vi "Parse.vi"(8 "Error In":errorcluster, 11 "object in":refnum<class "2022_5.lvclass">) -> (0 "Error Out":errorcluster, 3 "object out":refnum<class "2022_5.lvclass">)   [LabVIEW 2020, in "2022_5.lvclass"]
uses:
  2022_5.lvclass
  2022_5.lvclass/2022_5.ctl
  3533d167-0fa0-486d-894b-d8c4a5850acb.vi
  3533d167-0fa0-486d-894b-d8c4a5850acb.vi/be6f088c-3e4b-4523-ad48-2cdc85bad38a.vi
  3533d167-0fa0-486d-894b-d8c4a5850acb.vi/f202eadf-433e-4cdb-b986-b2351ce8d73c.vi
  3533d167-0fa0-486d-894b-d8c4a5850acb.vi/094751bc-bcf2-4346-afae-53942128b536.vi
panel:
  out "Stacks":cluster{"Crates":string[]}[](array[cluster])
  out "Stacks 2":string[][](array[string])
  out "Stacks":string[][](array[string])
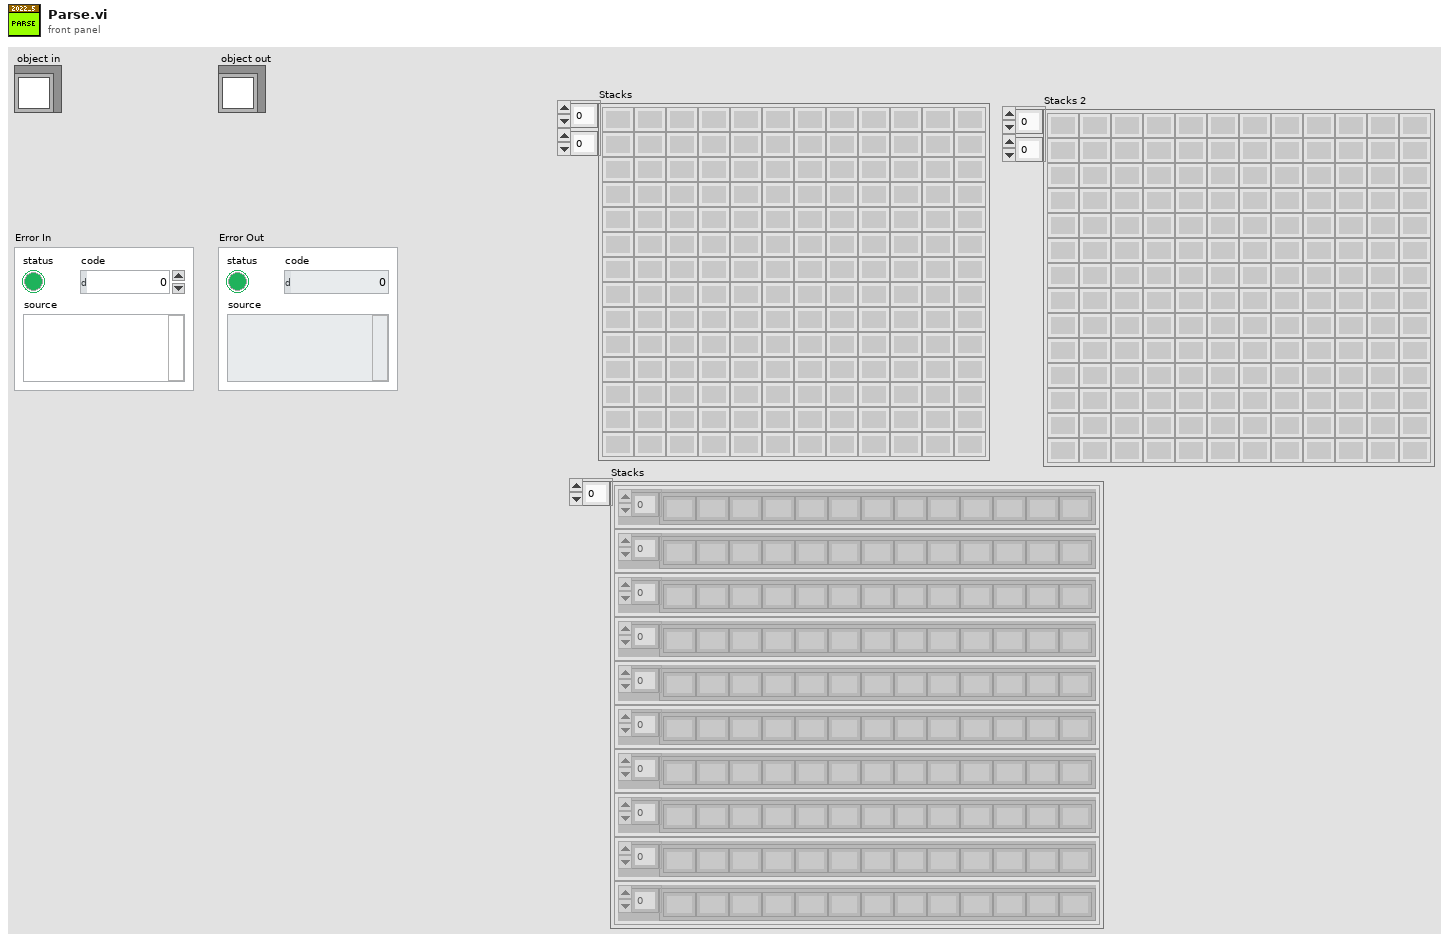
[diagram p1: front panel]
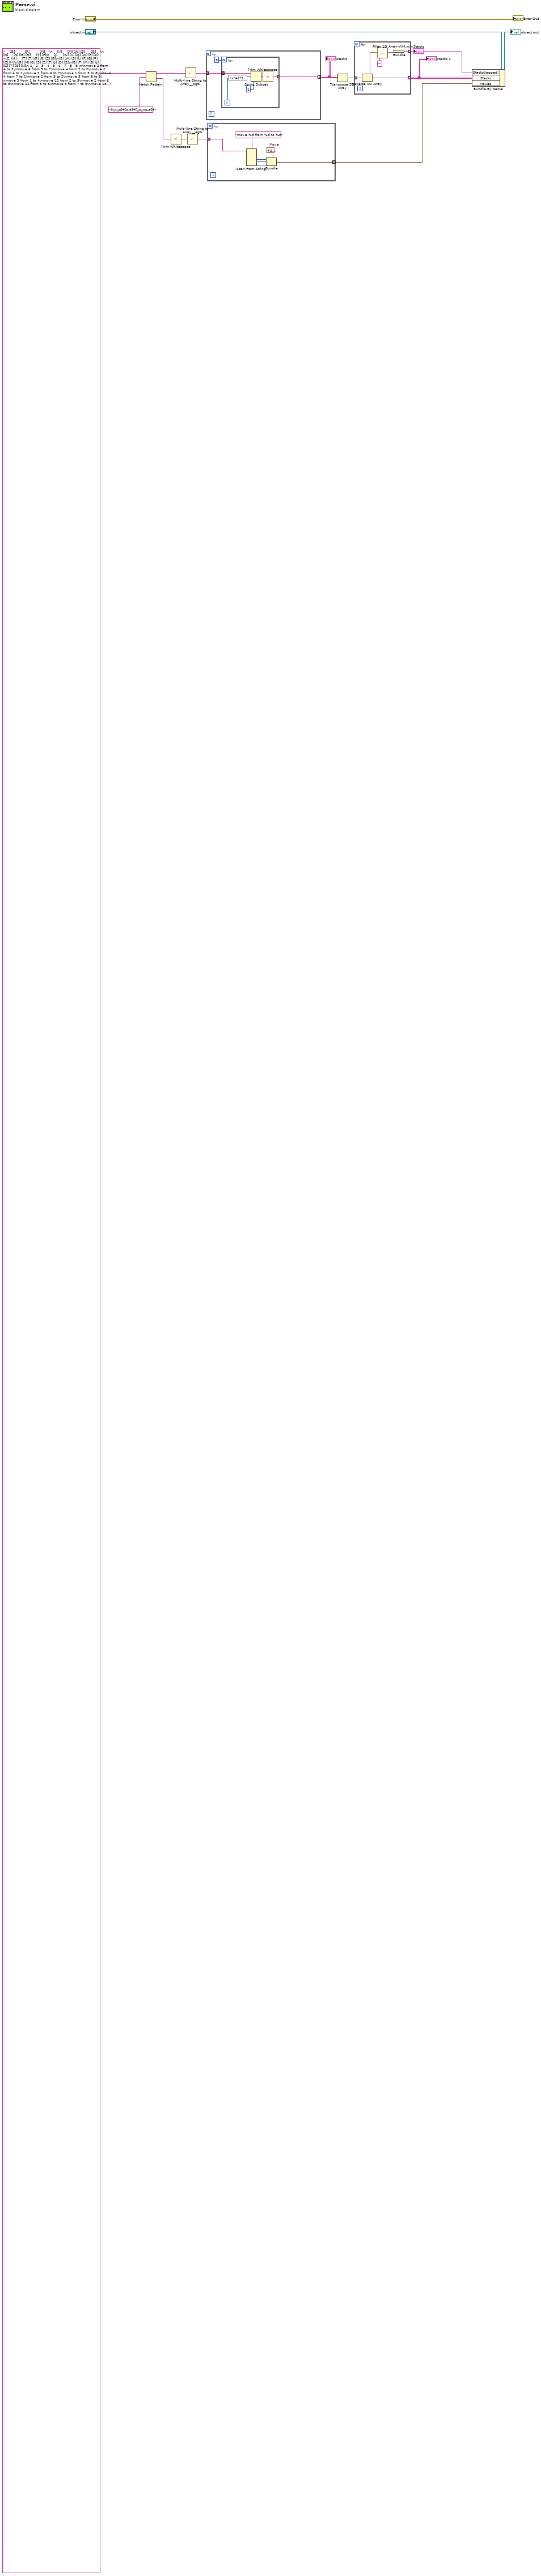
[diagram p0: block diagram]
diagram:
  n1 = Match Pattern(string="    [G]         [P]         [M]    \n    [V]     [M] [W] [S]     [Q]    \n    [N]     [N] [G] [H]     [T] [F]\n    [J]     [W] [V] [Q] [W] [F] [P]\n[C] [H]     [T] [T] [G] [B] [Z] [B]\n[S] [W] [S] [L] [F] [B] [P] [C] [H]\n[G] [M] [Q] [S] [Z] [T] [J] [D] [S]\n[B] [T] [M] [B] [J] [C] [T] [G] [N]\n 1   2   3   4   5   6   7   8   9 \n\nmove 2 from 4 to 2\nmove 6 from 9 to 7\nmove 4 from 7 to 2\nmove 2 from 4 to 1\nmove 2 from 6 to 7\nmove 1 from 3 to 8\nmove 4 from 7 to 1\nmove 2 from 3 to 2\nmove 3 from 8 to 5\nmove 3 from 1 to 4\nmove 12 from 2 to 5\nmove 2 from 6 to 8\nmove 12 from 5 to 8\nmove 3 from 7 to 9\nmove 18 from 8 to 9\nmove 2 from 8 to 6\nmove 3 from 2 to 3\nmove 14 from 9 to 4\nmove 1 from 1 to 3\nmove 7 from 9 to 3\nmove 1 from 2 to 1\nmove 8 from 4 to 5\nmove 5 from 6 to 3\nmove 2 from 7 to 9\nmove 3 from 4 to 9\nmove 4 from 9 to 6\nmove 4 from 6 to 1\nmove 8 from 4 to 6\nmove 10 from 1 to 2\nmove 13 from 3 to 2\nmove 17 from 5 to 9\nmove 2 from 5 to 1\nmove 9 from 9 to 7\nmove 1 from 3 to 6\nmove 2 from 1 to 8\nmove 11 from 2 to 4\nmove 5 from 6 to 8\nmove 1 from 6 to 3\nmove 1 from 1 to 4\nmove 3 from 8 to 6\nmove 3 from 2 to 8\nmove 9 from 7 to 9\nmove 4 from 4 to 7\nmove 1 from 9 to 5\nmove 15 from 9 to 7\nmove 7 from 8 to 3\nmove 1 from 5 to 6\nmove 2 from 6 to 9\nmove 8 from 2 to 6\nmove 3 from 4 to 3\nmove 1 from 2 to 5\nmove 4 from 9 to 3\nmove 1 from 3 to 4\nmove 13 from 6 to 2\nmove 1 from 5 to 1\nmove 4 from 4 to 9\nmove 6 from 3 to 2\nmove 11 from 2 to 7\nmove 6 from 3 to 4\nmove 3 from 3 to 2\nmove 1 from 3 to 4\nmove 1 from 1 to 3\nmove 3 from 9 to 2\nmove 1 from 3 to 1\nmove 4 from 7 to 1\nmove 1 from 9 to 5\nmove 5 from 1 to 4\nmove 11 from 2 to 4\nmove 1 from 5 to 3\nmove 1 from 2 to 3\nmove 12 from 4 to 2\nmove 2 from 7 to 2\nmove 7 from 4 to 3\nmove 5 from 4 to 1\nmove 7 from 7 to 6\nmove 4 from 1 to 8\nmove 1 from 8 to 5\nmove 8 from 3 to 2\nmove 4 from 7 to 4\nmove 13 from 7 to 1\nmove 2 from 8 to 6\nmove 5 from 4 to 9\nmove 1 from 3 to 6\nmove 1 from 5 to 8\nmove 1 from 2 to 9\nmove 4 from 2 to 6\nmove 2 from 8 to 6\nmove 10 from 1 to 3\nmove 4 from 9 to 4\nmove 2 from 1 to 3\nmove 5 from 2 to 9\nmove 4 from 9 to 2\nmove 1 from 1 to 2\nmove 13 from 2 to 4\nmove 15 from 4 to 5\nmove 3 from 6 to 8\nmove 8 from 3 to 8\nmove 1 from 4 to 2\nmove 14 from 5 to 1\nmove 1 from 5 to 4\nmove 1 from 4 to 2\nmove 8 from 6 to 7\nmove 3 from 6 to 2\nmove 2 from 9 to 1\nmove 8 from 8 to 7\nmove 9 from 1 to 5\nmove 7 from 5 to 3\nmove 14 from 7 to 9\nmove 2 from 2 to 3\nmove 7 from 2 to 1\nmove 1 from 6 to 1\nmove 4 from 9 to 2\nmove 8 from 3 to 6\nmove 2 from 4 to 3\nmove 4 from 3 to 5\nmove 5 from 5 to 7\nmove 2 from 6 to 9\nmove 6 from 6 to 2\nmove 4 from 2 to 3\nmove 1 from 6 to 2\nmove 2 from 7 to 8\nmove 13 from 9 to 5\nmove 2 from 7 to 1\nmove 14 from 1 to 5\nmove 15 from 5 to 7\nmove 3 from 8 to 7\nmove 5 from 3 to 5\nmove 6 from 5 to 7\nmove 4 from 1 to 7\nmove 1 from 2 to 5\nmove 3 from 2 to 8\nmove 11 from 5 to 2\nmove 10 from 7 to 1\nmove 1 from 3 to 4\nmove 10 from 2 to 9\nmove 1 from 5 to 8\nmove 6 from 7 to 3\nmove 1 from 4 to 6\nmove 2 from 3 to 8\nmove 1 from 2 to 1\nmove 4 from 3 to 9\nmove 3 from 1 to 6\nmove 2 from 7 to 1\nmove 1 from 5 to 6\nmove 1 from 3 to 8\nmove 4 from 1 to 4\nmove 5 from 2 to 9\nmove 3 from 1 to 4\nmove 18 from 9 to 7\nmove 4 from 8 to 4\nmove 3 from 1 to 2\nmove 1 from 9 to 7\nmove 1 from 4 to 7\nmove 1 from 6 to 2\nmove 1 from 2 to 5\nmove 25 from 7 to 3\nmove 7 from 4 to 2\nmove 8 from 7 to 9\nmove 4 from 8 to 6\nmove 1 from 8 to 5\nmove 4 from 6 to 5\nmove 2 from 9 to 5\nmove 3 from 5 to 8\nmove 4 from 6 to 4\nmove 12 from 3 to 5\nmove 11 from 3 to 2\nmove 13 from 5 to 8\nmove 4 from 9 to 6\nmove 7 from 4 to 9\nmove 2 from 6 to 2\nmove 12 from 2 to 7\nmove 1 from 6 to 3\nmove 1 from 5 to 6\nmove 2 from 5 to 3\nmove 15 from 8 to 6\nmove 4 from 6 to 7\nmove 1 from 5 to 1\nmove 10 from 2 to 8\nmove 8 from 8 to 3\nmove 8 from 6 to 8\nmove 2 from 7 to 6\nmove 9 from 9 to 7\nmove 8 from 8 to 9\nmove 1 from 1 to 3\nmove 1 from 2 to 7\nmove 7 from 3 to 1\nmove 3 from 8 to 5\nmove 3 from 1 to 6\nmove 7 from 9 to 2\nmove 2 from 3 to 7\nmove 5 from 7 to 9\nmove 17 from 7 to 5\nmove 2 from 7 to 6\nmove 10 from 6 to 3\nmove 1 from 1 to 3\nmove 6 from 9 to 3\nmove 1 from 2 to 9\nmove 2 from 7 to 9\nmove 2 from 9 to 7\nmove 1 from 5 to 8\nmove 1 from 8 to 5\nmove 6 from 2 to 5\nmove 1 from 6 to 1\nmove 5 from 3 to 5\nmove 1 from 6 to 8\nmove 1 from 7 to 9\nmove 2 from 9 to 3\nmove 15 from 5 to 2\nmove 2 from 1 to 8\nmove 2 from 3 to 7\nmove 2 from 8 to 3\nmove 3 from 5 to 9\nmove 1 from 8 to 6\nmove 1 from 9 to 6\nmove 3 from 7 to 6\nmove 17 from 3 to 4\nmove 1 from 1 to 2\nmove 6 from 2 to 9\nmove 16 from 4 to 1\nmove 4 from 6 to 8\nmove 9 from 5 to 6\nmove 8 from 6 to 2\nmove 2 from 9 to 5\nmove 2 from 3 to 5\nmove 1 from 6 to 2\nmove 1 from 4 to 8\nmove 14 from 1 to 3\nmove 8 from 5 to 3\nmove 20 from 3 to 1\nmove 1 from 8 to 2\nmove 1 from 9 to 6\nmove 1 from 6 to 7\nmove 1 from 7 to 3\nmove 22 from 1 to 2\nmove 3 from 3 to 6\nmove 27 from 2 to 8\nmove 2 from 2 to 8\nmove 2 from 6 to 9\nmove 2 from 9 to 4\nmove 2 from 4 to 8\nmove 1 from 1 to 3\nmove 14 from 8 to 5\nmove 1 from 3 to 9\nmove 3 from 9 to 2\nmove 5 from 2 to 8\nmove 10 from 2 to 9\nmove 1 from 6 to 7\nmove 1 from 7 to 5\nmove 7 from 5 to 2\nmove 2 from 9 to 2\nmove 1 from 6 to 2\nmove 2 from 9 to 5\nmove 3 from 5 to 6\nmove 6 from 5 to 3\nmove 1 from 5 to 6\nmove 4 from 3 to 9\nmove 2 from 9 to 8\nmove 3 from 9 to 5\nmove 23 from 8 to 1\nmove 2 from 6 to 1\nmove 1 from 5 to 7\nmove 2 from 3 to 5\nmove 2 from 9 to 5\nmove 4 from 9 to 7\nmove 2 from 9 to 4\nmove 1 from 5 to 4\nmove 5 from 8 to 5\nmove 2 from 6 to 2\nmove 3 from 7 to 3\nmove 1 from 3 to 4\nmove 3 from 2 to 8\nmove 4 from 1 to 6\nmove 2 from 6 to 3\nmove 4 from 1 to 2\nmove 3 from 8 to 1\nmove 13 from 2 to 5\nmove 4 from 3 to 2\nmove 14 from 5 to 7\nmove 5 from 2 to 7\nmove 18 from 7 to 9\nmove 4 from 4 to 7\nmove 2 from 5 to 4\nmove 17 from 9 to 5\nmove 1 from 9 to 1\nmove 1 from 7 to 2\nmove 5 from 7 to 2\nmove 18 from 1 to 4\nmove 1 from 7 to 3\nmove 1 from 3 to 6\nmove 2 from 1 to 3\nmove 1 from 6 to 5\nmove 2 from 6 to 8\nmove 1 from 8 to 9\nmove 1 from 8 to 3\nmove 13 from 4 to 5\nmove 1 from 1 to 6\nmove 3 from 2 to 4\nmove 1 from 6 to 1\nmove 3 from 2 to 9\nmove 3 from 3 to 1\nmove 5 from 4 to 5\nmove 30 from 5 to 3\nmove 1 from 4 to 6\nmove 1 from 9 to 8\nmove 1 from 9 to 6\nmove 21 from 3 to 7\nmove 3 from 1 to 6\nmove 1 from 1 to 4\nmove 1 from 9 to 6\nmove 1 from 8 to 2\nmove 1 from 3 to 6\nmove 1 from 9 to 3\nmove 5 from 4 to 8\nmove 1 from 2 to 4\nmove 9 from 5 to 7\nmove 2 from 5 to 9\nmove 2 from 8 to 2\nmove 2 from 6 to 3\nmove 1 from 4 to 1\nmove 4 from 3 to 8\nmove 2 from 9 to 2\nmove 4 from 2 to 6\nmove 1 from 1 to 4\nmove 2 from 6 to 9\nmove 2 from 5 to 4\nmove 1 from 3 to 1\nmove 1 from 1 to 3\nmove 2 from 9 to 1\nmove 5 from 3 to 5\nmove 1 from 1 to 8\nmove 4 from 6 to 4\nmove 5 from 5 to 6\nmove 18 from 7 to 5\nmove 1 from 3 to 4\nmove 12 from 7 to 5\nmove 15 from 5 to 6\nmove 1 from 5 to 8\nmove 1 from 3 to 7\nmove 1 from 1 to 2\nmove 1 from 2 to 4\nmove 1 from 7 to 9\nmove 2 from 8 to 2\nmove 1 from 2 to 4\nmove 4 from 4 to 2\nmove 1 from 2 to 1\nmove 1 from 9 to 8\nmove 4 from 6 to 4\nmove 3 from 2 to 6\nmove 1 from 2 to 6\nmove 8 from 4 to 3\nmove 1 from 1 to 3\nmove 6 from 6 to 1\nmove 1 from 3 to 6\nmove 5 from 1 to 7\nmove 10 from 5 to 9\nmove 3 from 9 to 8\nmove 7 from 6 to 2\nmove 1 from 7 to 8\nmove 3 from 5 to 8\nmove 3 from 6 to 2\nmove 6 from 8 to 9\nmove 1 from 5 to 3\nmove 2 from 3 to 1\nmove 2 from 4 to 8\nmove 6 from 6 to 9\nmove 1 from 1 to 4\nmove 17 from 9 to 2\nmove 1 from 4 to 1\nmove 2 from 7 to 8\nmove 1 from 9 to 8\nmove 3 from 8 to 4\nmove 3 from 1 to 4\nmove 9 from 8 to 2\nmove 1 from 8 to 4\nmove 12 from 2 to 7\nmove 4 from 7 to 4\nmove 1 from 8 to 1\nmove 10 from 4 to 2\nmove 3 from 3 to 2\nmove 1 from 9 to 7\nmove 11 from 7 to 3\nmove 1 from 3 to 1\nmove 2 from 3 to 9\nmove 1 from 3 to 7\nmove 2 from 1 to 9\nmove 1 from 6 to 5\nmove 7 from 3 to 6\nmove 1 from 7 to 3\nmove 3 from 3 to 4\nmove 1 from 5 to 7\nmove 2 from 4 to 3\nmove 2 from 4 to 8\nmove 1 from 7 to 6\nmove 2 from 6 to 8\nmove 1 from 9 to 2\nmove 1 from 9 to 5\nmove 1 from 5 to 1\nmove 1 from 8 to 6\nmove 1 from 3 to 2\nmove 4 from 6 to 1\nmove 5 from 1 to 4\nmove 11 from 2 to 4\nmove 2 from 8 to 2\nmove 1 from 8 to 9\nmove 27 from 2 to 5\nmove 4 from 6 to 3\nmove 3 from 2 to 4\nmove 2 from 5 to 9\nmove 1 from 5 to 7\nmove 2 from 9 to 5\nmove 14 from 4 to 7\nmove 2 from 4 to 7\nmove 3 from 4 to 8\nmove 4 from 3 to 1\nmove 4 from 1 to 8\nmove 2 from 3 to 9\nmove 2 from 9 to 3\nmove 7 from 8 to 9\nmove 1 from 3 to 8\nmove 2 from 3 to 2\nmove 25 from 5 to 9\nmove 1 from 5 to 8\nmove 1 from 8 to 7\nmove 26 from 9 to 1\nmove 23 from 1 to 5\nmove 7 from 9 to 7\nmove 1 from 9 to 8\nmove 1 from 9 to 2\nmove 5 from 7 to 1\nmove 20 from 5 to 6\nmove 1 from 7 to 6\nmove 2 from 5 to 3\nmove 1 from 8 to 6\nmove 21 from 6 to 8\nmove 1 from 6 to 4\nmove 1 from 1 to 7\nmove 2 from 1 to 6\nmove 1 from 1 to 3\nmove 1 from 2 to 5\nmove 1 from 2 to 6\nmove 2 from 7 to 6\nmove 6 from 7 to 9\nmove 3 from 1 to 2\nmove 17 from 8 to 1\nmove 1 from 4 to 1\nmove 2 from 6 to 9\nmove 3 from 8 to 9\nmove 2 from 3 to 7\nmove 2 from 9 to 8\nmove 4 from 7 to 3\nmove 4 from 3 to 4\nmove 2 from 5 to 8\nmove 4 from 8 to 4\nmove 3 from 6 to 8\nmove 18 from 1 to 5\nmove 1 from 3 to 4\nmove 3 from 2 to 4\nmove 5 from 9 to 1\nmove 10 from 7 to 5\nmove 5 from 1 to 3\nmove 5 from 3 to 5\nmove 5 from 4 to 3\nmove 2 from 4 to 2\nmove 5 from 8 to 3\nmove 25 from 5 to 2\nmove 3 from 3 to 6\nmove 1 from 1 to 3\nmove 3 from 6 to 7\nmove 1 from 4 to 2\nmove 1 from 5 to 8\nmove 2 from 4 to 9\nmove 1 from 8 to 1\nmove 20 from 2 to 7\nmove 10 from 7 to 1\nmove 1 from 1 to 7\nmove 4 from 7 to 8\nmove 5 from 5 to 4\nmove 4 from 8 to 6\nmove 1 from 1 to 3\nmove 5 from 7 to 4\nmove 2 from 1 to 5\nmove 4 from 9 to 1\nmove 3 from 2 to 5\nmove 5 from 5 to 1\nmove 1 from 9 to 1\nmove 11 from 1 to 3\nmove 1 from 6 to 2\nmove 7 from 3 to 5\nmove 11 from 3 to 7\nmove 1 from 2 to 6\nmove 7 from 7 to 8\nmove 1 from 9 to 1\nmove 2 from 3 to 1\nmove 1 from 5 to 3\nmove 4 from 1 to 6\nmove 4 from 6 to 3\nmove 9 from 4 to 5\nmove 2 from 8 to 2\nmove 4 from 6 to 9\nmove 3 from 2 to 4\nmove 1 from 8 to 6" ("PuzzleInput"), regular expression="[\\n\\s]+[0-9]+[\\s\\n0-9]+") -> (before substring=w10:string, after substring=w9:string)  [unwired: 1 in, 2 out]
  n2 = call <vilib>:"Trim Whitespace.vi"("string"=w9) -> ("trimmed string"=w5:string)  [unwired: 1 in]
  n3 = call <userlib>:"Multi-line String to Array__ogtk.vi"("string"=w10) -> ("lines"=w12:string[])
  n4 = call <userlib>:"Multi-line String to Array__ogtk.vi"("string"=w5) -> ("lines"=w8:string[])
  n5 = for {
    tunnel: w12 -> [w17] mode=indexing
    tunnel: [w16] -> w4 mode=indexing
    n6 = for {
      N: 9 -> [_]
      tunnel: w17 -> [w24]
      tunnel: [w19] -> w16 mode=indexing
      i -> [w22]
      n7 = expression code="(x*4)+1"(w22) -> (w23:i32)
      n8 = String Subset(string=w24, offset (0)=w23, length (rest)=1 ("length (rest)")) -> (substring=w20:string)
      n9 = call <vilib>:"Trim Whitespace.vi"("string"=w20) -> ("trimmed string"=w19:string)  [unwired: 1 in]
    }
  }
  "Stacks" <- w4
  n10 = for {
    tunnel: w8 -> [w30] mode=indexing
    tunnel: [w25] -> w6 mode=indexing
    w26 = cluster{"Qty":i32, "From":i32, "To":i32} {"Qty"=0, "From"=0, "To"=0}  # Move
    n11 = Scan From String(format string="move %d from %d to %d", input string=w30) -> (output 1=w29:i32, output 2=w28:i32, output 3=w27:i32)  [unwired: 5 in, 3 out]
    n12 = Bundle(cluster=w26, "Qty"=w29, "From"=w28, "To"=w27) -> (w25:cluster{"Qty":i32, "From":i32, "To":i32})
  }
  n13 = Transpose 2D Array(2D array=w4) -> (transposed array=w3:string[][])
  n14 = for {
    tunnel: w3 -> [w36] mode=indexing
    tunnel: [w35] -> w2 mode=indexing
    tunnel: [w32] -> w1 mode=indexing
    n15 = Reverse 1D Array(array=w36) -> (reversed array=w35:string[])
    n16 = call "Filter 1D Array-VIM.vim"("Item(s) to Filter"="", "Array"=w35) -> ("Filtered Array"=w33:string[])  [unwired: 5 in, 1 out]
    n17 = Bundle("Filtered Array"=w33) -> (w32:cluster{"Filtered Array":string[]})  [unwired: 1 in]
  }
  "Stacks 2" <- w2
  "Stacks" <- w1
  n18 = Bundle By Name(cluster="object in", "Stacks(Jagged)"=w1, "Stacks"=w2, "Moves"=w6) -> (→"object out":refnum<class "2022_5.lvclass">)
  "Error Out" <- "Error In"
